vi "Tool Object.vi"(8 "error in (no error)":errorcluster, 11 "Tool Funnel in":refnum<class "Tool Funnel.lvclass">) -> (0 "error out":errorcluster, 3 "Tool Funnel out":refnum<class "Tool Funnel.lvclass">)   [LabVIEW 2019, in "Tool Funnel.lvclass"]
uses:
  Tool Funnel.lvclass
  C:/Users/Albro/Documents/GitHub/AFM-Lithography/lvsrc/Classes/Tool/Tool Path/Tool Path.lvclass
  C:/Users/Albro/Documents/GitHub/AFM-Lithography/lvsrc/Classes/Tool/Tool Object/Tool Object.lvclass
  Settings/ObjectSettings/ObjectSettings.lvclass/ObjectSettings.ctl
  Settings/Funnel Settings/Funnel Settings.lvclass
  C:/Users/Albro/Documents/GitHub/AFM-Lithography/lvsrc/Classes/Settings/ObjectSettings/ObjectSettings.lvclass
  Parse/ParsePaths/Path.lvclass
  Tool Path/Tool Path.lvclass
  Tool Object/Tool Object.lvclass
  Settings/ObjectSettings/ObjectSettings.lvclass
panel:
  out "XY Graph":cluster{"X":dbl, "Y":dbl}[](graph)
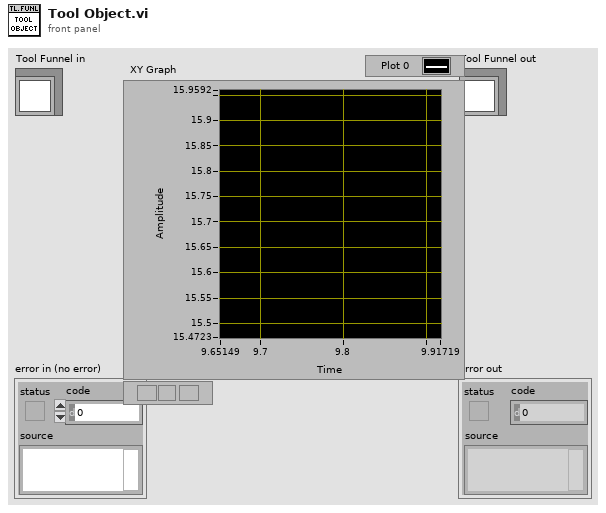
[diagram p1: front panel]
types:
  T1 = typedef "PathCommands.lvclass/Point.ctl" = cluster{"X":dbl, "Y":dbl}
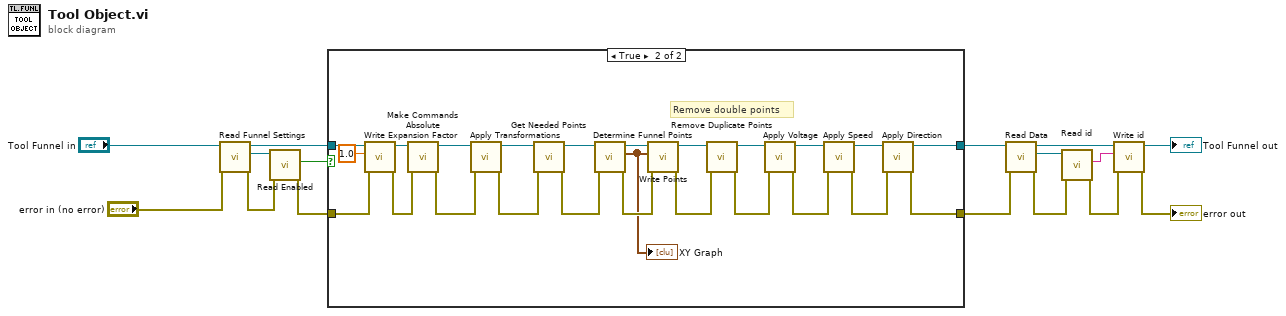
[diagram p0: block diagram]
diagram:
  n1 = call-dynamic "Read Funnel Settings.vi"("error in (no error)"="error in (no error)", "Tool Funnel in"="Tool Funnel in") -> ("error out"=w11:errorcluster, "Funnel Settings.lvclass"=w10:refnum<class "Funnel Settings.lvclass">, "Tool Funnel out"=w13:refnum<class "Tool Funnel.lvclass">)  [unwired: 7 in]
  n2 = call "Read Enabled.vi"("error in (no error)"=w11, "ObjectSettings in"=w10) -> ("error out"=w16:errorcluster, "Enabled"=w15:bool)  [unwired: 7 in, 1 out]
  n3 = case shown="True" w15 {
    tunnel: w13 -> [w18 w22]
    tunnel: [w18 w36] -> w4
    tunnel: w16 -> [w17 w20]
    tunnel: [w17 w37] -> w2
    frame False {
    }
    frame True {
      # "Remove double points"
      n4 = call-dynamic "Write Expansion Factor.vi"("error in (no error)"=w20, "Expansion Factor"=1.0, "Tool Path in"=w22) -> ("error out"=w21:errorcluster, "Tool Path out"=w23:refnum<class "Tool Funnel.lvclass">)  [unwired: 7 in]
      n5 = call "Make Commands Absolute.vi"("error in (no error)"=w21, "Tool Path in"=w23) -> ("error out"=w31:errorcluster, "Tool Path out"=w30:refnum<class "Tool Funnel.lvclass">)  [unwired: 8 in]
      n6 = call-dynamic "Apply Transformations.vi"("error in (no error)"=w31, "Tool Path in"=w30) -> ("error out"=w32:errorcluster, "Tool Path out"=w29:refnum<class "Tool Funnel.lvclass">)  [unwired: 8 in]
      n7 = call-dynamic "Get Needed Points.vi"("error in (no error)"=w32, "Tool Path in"=w29) -> ("error out"=w34:errorcluster, "Tool Path out"=w33:refnum<class "Tool Funnel.lvclass">)  [unwired: 8 in]
      n8 = call-dynamic "Determine Funnel Points.vi"("error in (no error)"=w34, "Tool Funnel in"=w33) -> ("error out"=w27:errorcluster, "Points"=w24:T1[], "Tool Funnel out"=w28:refnum<class "Tool Funnel.lvclass">)  [unwired: 7 in]
      "XY Graph" <- w24
      n9 = call-dynamic "Write Points.vi"("error in (no error)"=w27, "Points"=w24, "Tool Object in"=w28) -> ("error out"=w41:errorcluster, "Tool Object out"=w42:refnum<class "Tool Funnel.lvclass">)  [unwired: 7 in]
      n10 = call "Remove Duplicate Points.vi"("error in (no error)"=w41, "Tool Object in"=w42) -> ("error out"=w25:errorcluster, "Tool Object out"=w26:refnum<class "Tool Funnel.lvclass">)  [unwired: 8 in]
      n11 = call-dynamic "Apply Voltage.vi"("error in (no error)"=w25, "Tool Funnel in"=w26) -> ("error out"=w39:errorcluster, "Tool Funnel out"=w40:refnum<class "Tool Funnel.lvclass">)  [unwired: 8 in]
      n12 = call-dynamic "Apply Speed.vi"("error in (no error)"=w39, "Tool Funnel in"=w40) -> ("error out"=w38:errorcluster, "Tool Funnel out"=w35:refnum<class "Tool Funnel.lvclass">)  [unwired: 8 in]
      n13 = call-dynamic "Apply Direction.vi"("error in (no error)"=w38, "Tool Funnel in"=w35) -> ("error out"=w37:errorcluster, "Tool Funnel out"=w36:refnum<class "Tool Funnel.lvclass">)  [unwired: 8 in]
    }
  }
  n14 = call-dynamic "Read Data.vi"("error in (no error)"=w2, "Tool Path in"=w4) -> ("error out"=w6:errorcluster, "Path.lvclass"=w9:refnum<class "Path.lvclass">, "Tool Path out"=w8:refnum<class "Tool Funnel.lvclass">)  [unwired: 7 in]
  n15 = call-dynamic "Read id.vi"("error in (no error)"=w6, "SVG Object in"=w9) -> ("error out"=w5:errorcluster, "id"=w7:string)  [unwired: 7 in, 1 out]
  n16 = call-dynamic "Write id.vi"("error in (no error)"=w5, "id"=w7, "Tool Path in"=w8) -> ("error out"=→"error out":errorcluster, "Tool Path out"=→"Tool Funnel out":refnum<class "Tool Funnel.lvclass">)  [unwired: 7 in]
